vi "Open Control by Reference.vi"(8 "error in (no error)":errorcluster, 10 "VI Description in":string, 11 "ctl path":path) -> (0 "error out":errorcluster, 2 "VI Description":string, 3 "Value":variant)   [LabVIEW 2019, in "JSON-Schema.lvlib"]
uses:
  JSON-Schema.lvlib
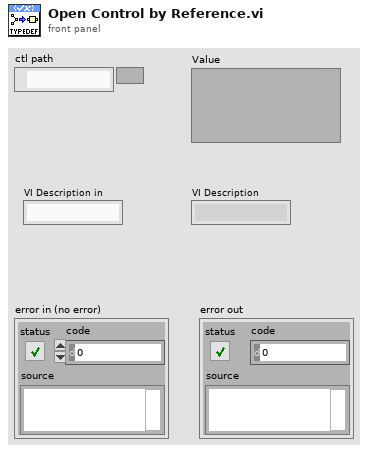
[diagram p1: front panel]
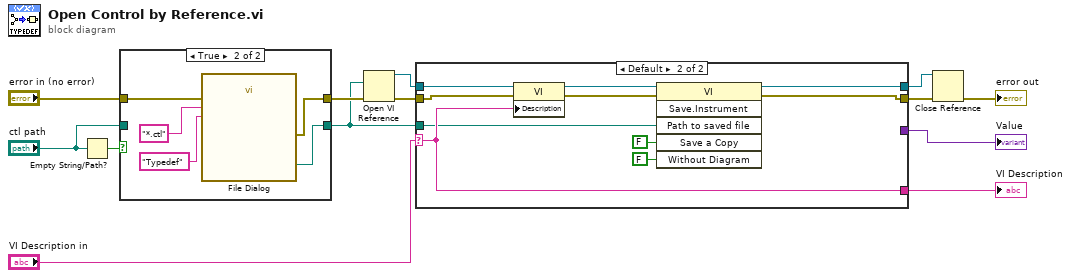
[diagram p0: block diagram]
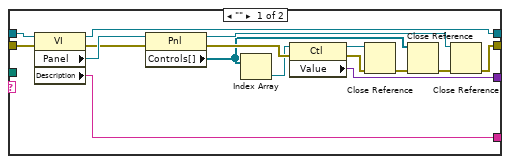
[diagram p2: hidden frame]
diagram:
  n1 = Empty String/Path?(string/path="ctl path") -> (empty?=w9:bool)
  n2 = case shown="True" w9 {
    tunnel: [w15 w20] -> w2
    tunnel: "error in (no error)" -> [w14 w19]
    tunnel: [w14 w18] -> w10
    tunnel: "ctl path" -> [w15 _]
    frame False {
    }
    frame True {
      n3 = call "File Dialog"("error in"=w19, "pattern (all files)"="*.ctl", "pattern label"="Typedef") -> ("selected path"=w20:path, "error out"=w18:errorcluster)  [unwired: 9 in, 2 out]
    }
  }
  n4 = Open VI Reference(vi path=w2, error in (no error)=w10) -> (vi reference=w13:refnum<vi>, error out=w12:errorcluster)  [unwired: 4 in]
  n5 = case shown="Default" "VI Description in" {
    selector: "VI Description in" -> [_ w44]
    tunnel: w13 -> [w36 w46]
    tunnel: w12 -> [w35 w45]
    tunnel: [w21 w41] -> w3
    tunnel: [w34 w44] -> w8
    tunnel: [w23 _] -> w6
    tunnel: [w22 w40] -> w5
    tunnel: w2 -> [_ w39]
    frame "" {
      n6 = property class="VI"(reference=w36, error in=w35) -> (reference out=w22:refnum<vi>, error out=w24:errorcluster, "Panel"=w25:refnum<vi>, "Description"=w34:string)
      n7 = property class="Pnl"(reference=w25, error in=w24) -> (reference out=w27:refnum<vi>, error out=w33:errorcluster, "Controls[]"=w26:refnum<vi>[])
      n8 = Index Array(array=w26) -> (element=w28:refnum<vi>)  [unwired: 1 in]
      n9 = property class="Ctl"(reference=w28, error in=w33) -> (reference out=w30:refnum<vi>, error out=w32:errorcluster, "Value"=w23:variant)
      n10 = Close Reference(reference=w30, error in (no error)=w32) -> (error out=w31:errorcluster)
      n11 = Close Reference(reference=w26, error in (no error)=w31) -> (error out=w29:errorcluster)
      n12 = Close Reference(reference=w27, error in (no error)=w29) -> (error out=w21:errorcluster)
    }
    frame Default {
      n13 = property class="VI"(reference=w46, error in=w45, "Description"=w44) -> (reference out=w43:refnum<vi>, error out=w42:errorcluster)
      n14 = invoke class="VI" method="Save.Instrument"(reference=w43, error in=w42, "Path to saved file"=w39, "Save a Copy"=FALSE, "Without Diagram"=FALSE) -> (reference out=w40:refnum<vi>, error out=w41:errorcluster)  [unwired: 1 in, 4 out]
    }
  }
  "Value" <- w6
  "VI Description" <- w8
  n15 = Close Reference(reference=w5, error in (no error)=w3) -> (error out=→"error out":errorcluster)
